vi "LM model function and gradient (1-Exp, Convolved) v2.vi"(3 "output control":T1, 4 "data":variant, 5 "X":dbl[](array[numeric]), 6 "a":dbl[](array[numeric])) -> (0 "error out":errorcluster, 1 "f'(X,a)":dbl[][](array[numeric]), 2 "f(X,a)":dbl[](array[numeric]))   [LabVIEW 2021, in "Fits.lvlib"]
doc: "This template is the starting point for creating a model function to be passed to the Nonlinear Curve Fit.vi."
uses:
  Fits.lvlib
  <vilib>/gmath/NumericalOptimization/LM_output select.ctl
  <vilib>/Analysis/2dsp.llb/1D Convolution (DBL).vi
  1e868266-4877-41c0-b2cd-7e3a67bf7ec7.vi
  <vilib>/Analysis/NI_AALPro.lvlib
  Arrays/Arrays.lvlib
  Error/Error.lvlib
  <vilib>/gmath/NI_Gmath.lvlib
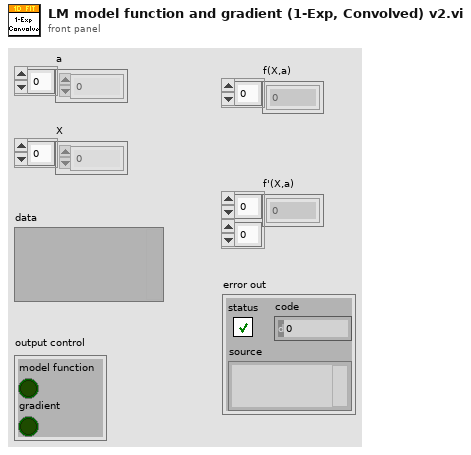
[diagram p1: front panel]
types:
  T1 = typedef "NI_Gmath.lvlib/LM_output select.ctl" = cluster{"model function":bool, "gradient":bool}
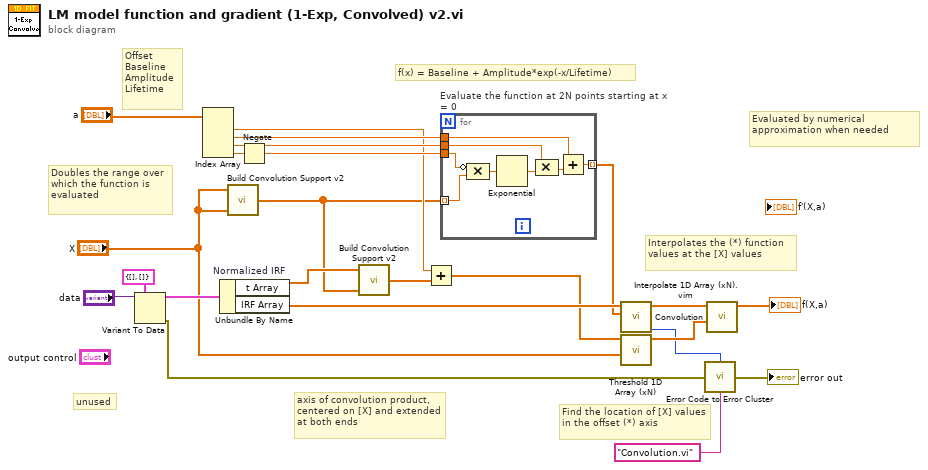
[diagram p0: block diagram]
diagram:
  # "Doubles the range over which the function is evaluated"
  # "unused"
  # "Evaluated by numerical approximation when needed"
  # "Interpolates the (*) function values at the [X] values"
  # "Find the location of [X] values in the offset (*) axis"
  # "axis of convolution product, centered on [X] and extended at both ends"
  # "f(x) = Baseline + Amplitude*exp(-x/Lifetime)"
  # "Offset\nBaseline\nAmplitude\nLifetime"
  n1 = Variant To Data(type=cluster{"t Array":dbl[], "IRF Array":dbl[]} {"t Array"=[], "IRF Array"=[]} ("IRF"), Variant="data") -> (data=w17:cluster{"t Array":dbl[], "IRF Array":dbl[]}, error out=w4:errorcluster)  [unwired: 1 in]
  n2 = Index Array(array="a") -> (element #1=w9:dbl, element #2=w20:dbl, element #3=w19:dbl, element #4=w21:dbl)  [unwired: 4 in]
  n3 = Unbundle By Name "Normalized IRF"(w17) -> ("t Array"=w12:dbl[], "IRF Array"=w16:dbl[])
  n4 = call "Build Convolution Support v2.vi"("X Array 2"="X", "X Array 1"="X") -> ("X Arrays Convolution Support"=w6:dbl[])  [unwired: 3 in]
  n5 = Negate(x=w21) -> (-x=w10:dbl)
  n6 = call "Build Convolution Support v2.vi"("X Array 2"=w6, "X Array 1"=w12) -> ("X Arrays Convolution Support"=w11:dbl[])  [unwired: 3 in]
  n7 = Add(x=w9, y=w11) -> (x+y=w8:dbl[])
  n8 = for "Evaluate the function at 2N points starting at x = 0" {
    tunnel: w10 -> [w31]
    tunnel: w20 -> [w30]
    tunnel: w19 -> [w29]
    tunnel: [w25] -> w15 mode=indexing
    tunnel: w6 -> [w24] mode=indexing
    n9 = Compound Arithmetic op=MULTIPLY(invert w31, w24) -> (w28:dbl)
    n10 = Exponential(1:w28) -> (0:w27:dbl)
    n11 = Compound Arithmetic op=MULTIPLY(w29, w27) -> (w26:dbl)
    n12 = Add(x=w30, y=w26) -> (x+y=w25:dbl)
  }
  n13 = call-poly <vilib>:"Convolution.vi"("Y"=w15, "X"=w16) -> ("error"=w2:i32, "X * Y"=w7:dbl[])  [unwired: 8 in]
  n14 = call "Threshold 1D Array (xN).vi"("Search Values"="X", "X"=w8) -> ("Interpolated Indices"=w13:dbl[])  [unwired: 9 in]
  n15 = call "Error Code to Error Cluster.vi"("Error Code"=w2, "Error Source"="Convolution.vi", "Error In"=w4) -> ("Error Out"=→"error out":errorcluster)  [unwired: 12 in]
  n16 = call "Interpolate 1D Array (xN).vim"("Interpolated Indices"=w13, "Y"=w7) -> ("Interpolated Y"=→"f(X,a)":dbl[])  [unwired: 9 in]
